vi "test_MonoMirrorPosition.vi"(8 "error in":errorcluster, 11 "Monochromator in":refnum<class "Monochromator.lvclass">) -> (0 "error out":errorcluster, 3 "Monochromator out":refnum<class "Monochromator.lvclass">)   [LabVIEW 2023, in "horiba.test.lvlib"]
uses:
  horiba.test.lvlib
  Classes/Mono/Monochromator.lvclass
  <vilib>/addons/_JKI Toolkits/Caraya/classes/Assert/Assert Equal Value_Variant.vi
  <vilib>/addons/_JKI Toolkits/Caraya/classes/Test/Test.lvclass
  <vilib>/addons/_JKI Toolkits/Caraya/classes/Assert/Assert.lvclass
  <userlib>/_OpenG.lib/lvdata/lvdata.llb/openg_variant.lvlib
panel:
  # "Connector Pane"
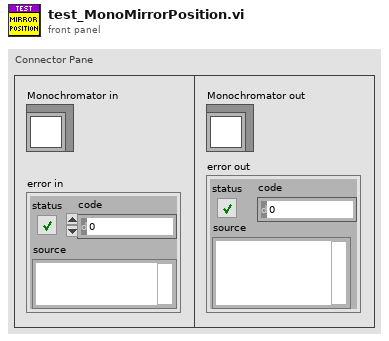
[diagram p1: front panel]
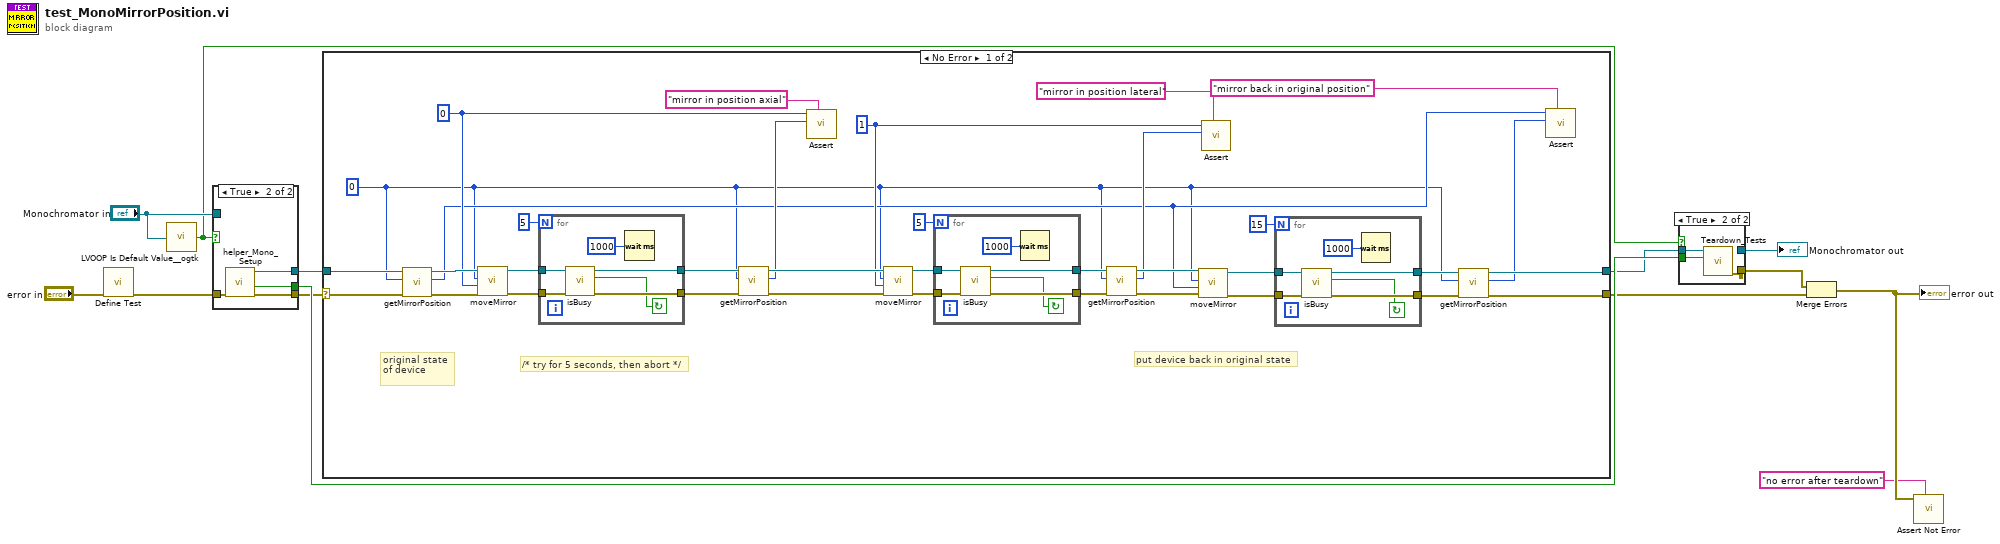
[diagram p0: block diagram]
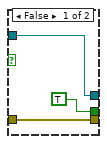
[diagram p2: hidden frame]
diagram:
  n1 = call <vilib>:"Define Test.vi"("error in (no error)"="error in") -> ("error out"=w7:errorcluster)  [unwired: 9 in, 1 out]
  n2 = call <userlib>:"LVOOP Is Default Value__ogtk.vi"("Object"="Monochromator in") -> ("Is Default Value?"=w8:bool)
  n3 = case shown="True" w8 {
    tunnel: w7 -> [w15 w20]
    tunnel: [w15 w19] -> w2
    tunnel: [w16 w18] -> w5
    tunnel: [TRUE ("Module Was Already Running?") w17] -> w10
    tunnel: "Monochromator in" -> [w16 _]
    frame False {
    }
    frame True {
      n4 = call "helper_Mono_Setup.vi"("error in"=w20) -> ("error out"=w19:errorcluster, "Module Was Already Running?"=w17:bool, "Monochromator out"=w18:refnum<class "Monochromator.lvclass">)  [unwired: 7 in, 1 out]
    }
  }
  n5 = case shown="No Error" w2 {
    selector: w2 -> [w37 w75]
    tunnel: [w34 w74] -> w4
    tunnel: w5 -> [w36 w74]
    tunnel: [w35 w75] -> w1
    frame No Error {
      w26 = 1
      w28 = 0
      w21 = 0 ("locationId")
      # "/* try for 5 seconds, then abort */"
      # "put device back in original state"
      # "original state of device"
      n6 = call "getMirrorPosition.vi"("error in (no error)"=w37, "locationId"=w21, "Monochromator in"=w36) -> ("error out"=w54:errorcluster, "position"=w22:i32, "Monochromator out"=w55:refnum<class "Monochromator.lvclass">)  [unwired: 6 in]
      n7 = call "moveMirror.vi"("error in (no error)"=w54, "position"=w28, "locationId"=w21, "Monochromator in"=w55) -> ("error out"=w47:errorcluster, "Monochromator out"=w49:refnum<class "Monochromator.lvclass">)  [unwired: 4 in, 2 out]
      n8 = for {
        N: 5 -> [_]
        tunnel: w49 -> [w66]
        tunnel: [w65] -> w48
        tunnel: w47 -> [w64]
        tunnel: [w63] -> w46
        stop <- w62 continue-if-true
        n9 = call "isBusy.vi"("error in (no error)"=w64, "Monochromator in"=w66) -> ("error out"=w63:errorcluster, "mono is busy?"=w62:bool, "Monochromator out"=w65:refnum<class "Monochromator.lvclass">)  [unwired: 7 in]
        n10 = Wait (ms)(milliseconds to wait=u32 1000) -> ()  [unwired: 1 out]
      }
      n11 = call "getMirrorPosition.vi"("error in (no error)"=w46, "locationId"=w21, "Monochromator in"=w48) -> ("error out"=w52:errorcluster, "position"=w29:i32, "Monochromator out"=w53:refnum<class "Monochromator.lvclass">)  [unwired: 6 in]
      n12 = call-poly <vilib>:"Assert.vi"("Label"="mirror in position axial", "Y"=w29, "X"=w28) -> ()  [unwired: 7 in, 2 out]
      n13 = call "moveMirror.vi"("error in (no error)"=w52, "position"=w26, "locationId"=w21, "Monochromator in"=w53) -> ("error out"=w43:errorcluster, "Monochromator out"=w45:refnum<class "Monochromator.lvclass">)  [unwired: 4 in, 2 out]
      n14 = for {
        N: 5 -> [_]
        tunnel: w45 -> [w60]
        tunnel: [w59] -> w44
        tunnel: w43 -> [w58]
        tunnel: [w57] -> w42
        stop <- w56 continue-if-true
        n15 = call "isBusy.vi"("error in (no error)"=w58, "Monochromator in"=w60) -> ("error out"=w57:errorcluster, "mono is busy?"=w56:bool, "Monochromator out"=w59:refnum<class "Monochromator.lvclass">)  [unwired: 7 in]
        n16 = Wait (ms)(milliseconds to wait=u32 1000) -> ()  [unwired: 1 out]
      }
      n17 = call "getMirrorPosition.vi"("error in (no error)"=w42, "locationId"=w21, "Monochromator in"=w44) -> ("error out"=w50:errorcluster, "position"=w25:i32, "Monochromator out"=w51:refnum<class "Monochromator.lvclass">)  [unwired: 6 in]
      n18 = call "moveMirror.vi"("error in (no error)"=w50, "position"=w22, "locationId"=w21, "Monochromator in"=w51) -> ("error out"=w39:errorcluster, "Monochromator out"=w41:refnum<class "Monochromator.lvclass">)  [unwired: 4 in, 2 out]
      n19 = call-poly <vilib>:"Assert.vi"("Label"="mirror in position lateral", "Y"=w25, "X"=w26) -> ()  [unwired: 7 in, 2 out]
      n20 = for {
        N: 15 -> [_]
        tunnel: w41 -> [w72]
        tunnel: [w71] -> w40
        tunnel: w39 -> [w70]
        tunnel: [w69] -> w38
        stop <- w68 continue-if-true
        n21 = call "isBusy.vi"("error in (no error)"=w70, "Monochromator in"=w72) -> ("error out"=w69:errorcluster, "mono is busy?"=w68:bool, "Monochromator out"=w71:refnum<class "Monochromator.lvclass">)  [unwired: 7 in]
        n22 = Wait (ms)(milliseconds to wait=u32 1000) -> ()  [unwired: 1 out]
      }
      n23 = call "getMirrorPosition.vi"("error in (no error)"=w38, "locationId"=w21, "Monochromator in"=w40) -> ("error out"=w35:errorcluster, "position"=w23:i32, "Monochromator out"=w34:refnum<class "Monochromator.lvclass">)  [unwired: 6 in]
      n24 = call-poly <vilib>:"Assert.vi"("Label"="mirror back in original position", "Y"=w23, "X"=w22) -> ()  [unwired: 7 in, 2 out]
    }
    frame Error {
    }
  }
  n25 = case shown="True" w8 {
    tunnel: w4 -> [w76 w79]
    tunnel: [_ w78] -> w6
    tunnel: w10 -> [_ w77]
    tunnel: [w76 _] -> w3
    frame False {
    }
    frame True {
      n26 = call "Teardown_Tests.vi"("Module Was Already Running?"=w77, "horiba.lvlib:GenericDevice"=w79) -> ("error out"=w78:errorcluster)  [unwired: 8 in, 1 out]
    }
  }
  "Monochromator out" <- w3
  n27 = Merge Errors(w6, w1) -> (w12:errorcluster)
  "error out" <- w12
  n28 = call <vilib>:"Assert Not Error.vi"("Label"="no error after teardown", "Not Error?"=w12) -> ()  [unwired: 8 in, 2 out]
